vi "Exp no 5b Gray to Binary Conversion.vi"() -> ()   [LabVIEW 2010]
panel:
  out "B4":bool
  out "B3":bool
  out "B2":bool
  out "B1":bool
  in  "G4":bool
  in  "G3":bool
  in  "G2":bool
  in  "G1":bool
  # "GRAY CODE TO BINARY CODE CONVERSION"
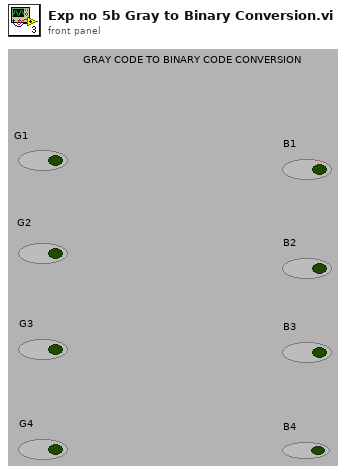
[diagram p1: front panel]
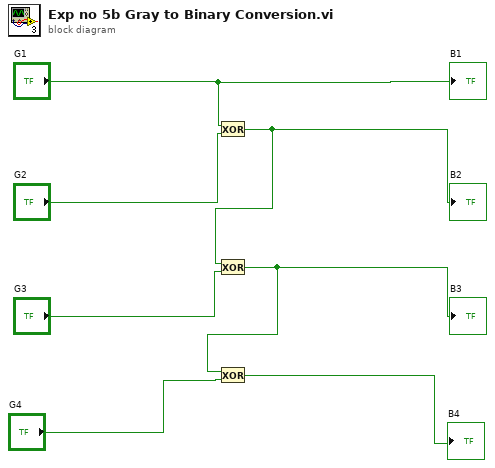
[diagram p0: block diagram]
diagram:
  n1 = Exclusive Or(1:"G2", 2:"G1") -> (0:w5:bool)
  "B2" <- w5
  n2 = Exclusive Or(1:"G3", 2:w5) -> (0:w3:bool)
  "B3" <- w3
  n3 = Exclusive Or(1:"G4", 2:w3) -> (0:→"B4":bool)
  "B1" <- "G1"
